vi "System Options.vi"(6 "Enable Mouse Lock (Disable)":bool, 7 "Enable Keyboard Lock (Disable)":bool, 8 "error in (no error)":errorcluster, 9 "Enable Beep For Warning (Disable)":bool, 10 "Enable Beep For Operation Complete (Enable)":bool=TRUE, 11 "VISA resource name":refnum<visa-resource-name>) -> (0 "error out":errorcluster, 3 "VISA resource name out":refnum<visa-resource-name>)   [LabVIEW 2011, in "Agilent E5052X.lvlib"]
doc: "Sets system options for the instrument. \n\n<b>Note: </b>\n\nSystem options that can be set are for the beeper, mouse and the keyboard."
uses:
  Agilent E5052X.lvlib
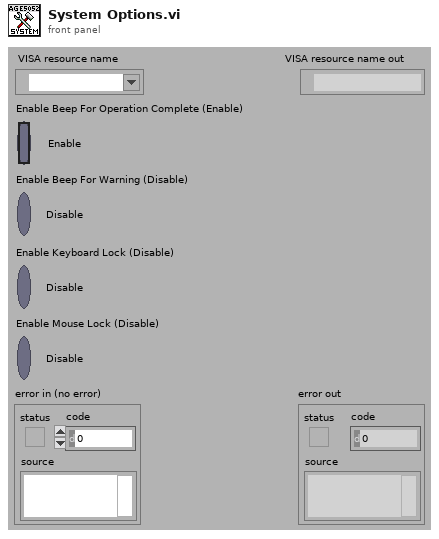
[diagram p1: front panel]
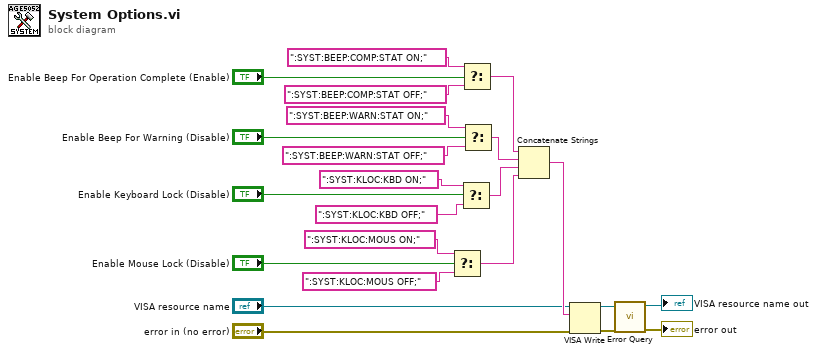
[diagram p0: block diagram]
diagram:
  n1 = Select(t=":SYST:KLOC:MOUS ON;", s="Enable Mouse Lock (Disable)", f=":SYST:KLOC:MOUS OFF;") -> (s? t:f=w1:string)
  n2 = Select(t=":SYST:KLOC:KBD ON;", s="Enable Keyboard Lock (Disable)", f=":SYST:KLOC:KBD OFF;") -> (s? t:f=w2:string)
  n3 = Select(t=":SYST:BEEP:COMP:STAT ON;", s="Enable Beep For Operation Complete (Enable)", f=":SYST:BEEP:COMP:STAT OFF;") -> (s? t:f=w4:string)
  n4 = Select(t=":SYST:BEEP:WARN:STAT ON;", s="Enable Beep For Warning (Disable)", f=":SYST:BEEP:WARN:STAT OFF;") -> (s? t:f=w3:string)
  n5 = Concatenate Strings(w4, w3, w2, w1) -> (w23:string)
  n6 = VISA Write(VISA resource name="VISA resource name", write buffer=w23, error in (no error)="error in (no error)") -> (VISA resource name out=w20:refnum<visa-resource-name>, error out=w19:errorcluster)  [unwired: 1 out]
  n7 = call "Error Query.vi"("error in (no error)"=w19, "VISA resource name"=w20) -> ("error out"=→"error out":errorcluster, "VISA resource name out"=→"VISA resource name out":refnum<visa-resource-name>)  [unwired: 6 in, 2 out]
